vi "LIN_SignalValue_Conver_Physical.vi"(10 "FDatas":u8[](array[numeric]), 11 "TLINSignal":T1) -> (3 "Signal Value":dbl)   [LabVIEW 2014]
uses:
  Typedef/LIN/TLINSignal.ctl
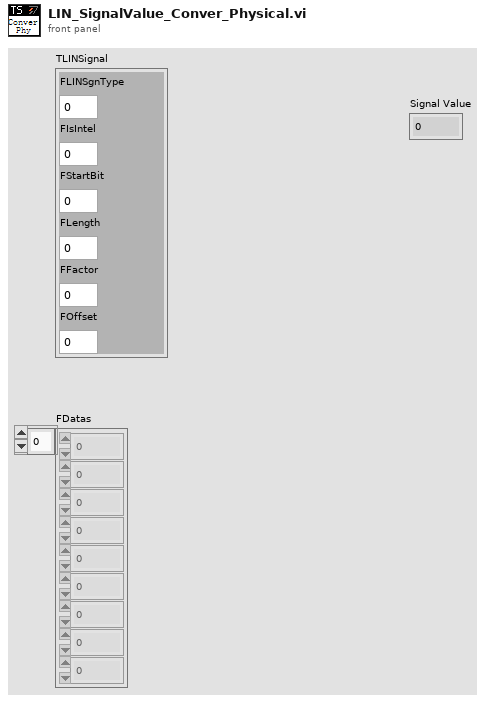
[diagram p1: front panel]
types:
  T1 = typedef "TLINSignal.ctl" = cluster{"FLINSgnType":u8, "FIsIntel":u8, "FStartBit":i32, "FLength":i32, "FFactor":dbl, "FOffset":dbl}
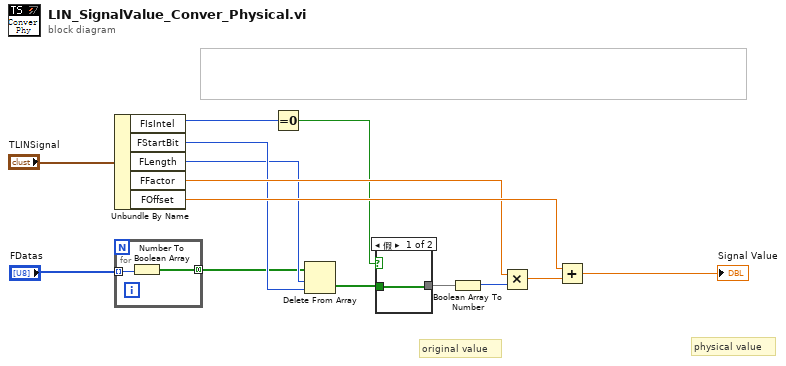
[diagram p0: block diagram]
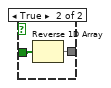
[diagram p2: hidden frame]
diagram:
  # "physical value"
  # "original value"
  n1 = Unbundle By Name("TLINSignal") -> ("FIsIntel"=w7:u8, "FStartBit"=w6:i32, "FLength"=w5:i32, "FFactor"=w11:dbl, "FOffset"=w13:dbl)
  n2 = for {
    tunnel: "FDatas" -> [w16] mode=indexing
    tunnel: [w15] -> w4 mode=concatenating
    n3 = Number To Boolean Array(number=w16) -> (Boolean array=w15:bool[])
  }
  n4 = Equal To 0?(x=w7) -> (x = 0?=w8:bool)
  n5 = Delete From Array(array=w4, length=w5, index=w6) -> (deleted portion=w1:bool[])  [unwired: 1 out]
  n6 = case shown="假" w8 {
    tunnel: w1 -> [w17 w19]
    tunnel: [w17 w18] -> w9
    frame False {
    }
    frame True {
      n7 = Reverse 1D Array(array=w19) -> (reversed array=w18:bool[])
    }
  }
  n8 = Boolean Array To Number(Boolean array=w9) -> (number=w10:u32)
  n9 = Multiply(x=w11, y=w10) -> (x*y=w12:dbl)
  n10 = Add(x=w13, y=w12) -> (x+y=→"Signal Value":dbl)
